vi "core_wait_for_notification.vi"(6 "ignore previous (T)":bool=TRUE, 8 "Error in":errorcluster caption="Error in (no error)", 10 "notifier":T1) -> (0 "Error out":errorcluster, 2 "notifier duplicate":T1, 4 "notification":bool)   [LabVIEW 2015]
uses:
  boolean_notifier.ctl
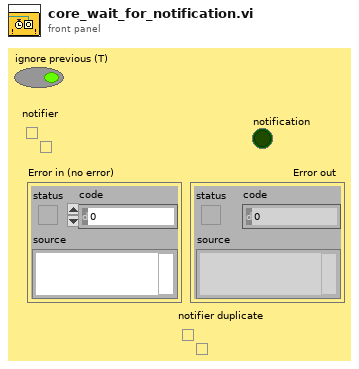
[diagram p1: front panel]
types:
  T1 = typedef "boolean_notifier.ctl" = refnum<notifier>
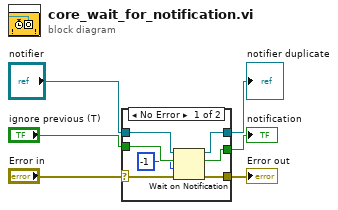
[diagram p0: block diagram]
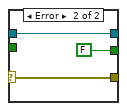
[diagram p2: hidden frame]
diagram:
  n1 = case shown="No Error" "Error in" {
    selector: "Error in" -> [w11 w16]
    tunnel: "ignore previous (T)" -> [w12 _]
    tunnel: [w10 w16] -> w4
    tunnel: "notifier" -> [w13 w15]
    tunnel: [w9 w15] -> w1
    tunnel: [w8 FALSE] -> w3
    frame No Error {
      n2 = Wait on Notification(notifier=w13, ignore previous (F)=w12, timeout in ms (-1)=-1 ("ms timeout (-1)"), error in (no error)=w11) -> (notifier out=w9:T1, notification=w8:bool, error out=w10:errorcluster)  [unwired: 1 out]
    }
    frame Error {
    }
  }
  "Error out" <- w4
  "notification" <- w3
  "notifier duplicate" <- w1
